vi "Aquisição.vi"(8 "error in (no error)":errorcluster, 10 "rt fifo":refnum<k33>, 11 "FPGA VI Reference In":refnum<k20>) -> (0 "error out":errorcluster, 2 "rt fifo 2":refnum<k33>, 3 "FPGA VI Reference Out":refnum<k20>)   [LabVIEW 2013]
uses:
  PRBScontrol.ctl
  <vilib>/Platform/TimedLoop/XDataNode/timing_clust.ctl
  <vilib>/Platform/TimedLoop/XDataNode/nitl_modes.ctl
  <vilib>/Platform/TimedLoop/XDataNode/wakeup.ctl
  PRBSparameters.ctl
  <vilib>/rvi/interface/common/niFpgaWaitOnOcc.vi
  <vilib>/Utility/error.llb/Error Cluster From Error Code.vi
  <vilib>/rvi/errors/niLvFpgaAdjustHostInterfaceError.vi
  <vilib>/Platform/TimedLoop/XDataNode/XDataNode.xnode
  <vilib>/rvi/interface/nirviReadWriteControl/nirviReadWriteControl.xnode
  <vilib>/Platform/TimedLoop/XDataNode/XDNodeRunTimeDep.lvlib
  NiFpgaLv.dll
  <vilib>/rvi/interface/Simulation/niFpgaSimulationCallBeginRW.vi
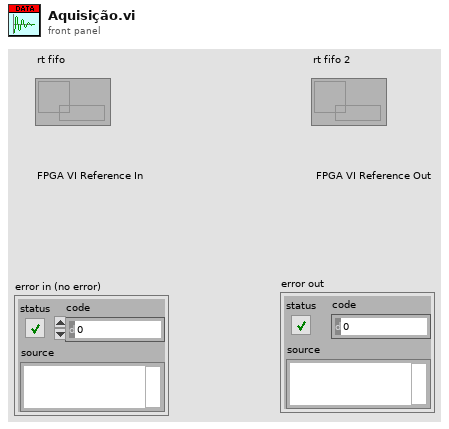
[diagram p1: front panel]
types:
  T1 = typedef "PRBScontrol.ctl" = enum16{"Create", "Get data point"}
  T2 = typedef "XDNodeRunTimeDep.lvlib/timing_clust.ctl" = cluster{"Expected End [f-1]":u64, "Actual End [f-1]":u64, "Finished Late? [f-1]":bool, "Expected End [i-1]":u64, "Actual End [i-1]":u64, "Finished Late? [i-1]":bool, "Expected Start [i]":u64, "Actual Start [i]":u64, "Expected Start [f]":u64, "Actual Start [f]":u64, "Source Name":string, "Structure Name":string, "Period":i64, "Deadline":i64, "Offset":i64, "Start":i64, "Priority":i32, "Timeout":i32, "Mode":T3, "Wakeup Reason":T4, "Error":errorcluster, "Source Type":string, "Secondary Source Type":string, "Global End Time":u64, "Global Start Time":u64, "Frame Duration":u64, "Iteration Duration":u64, "Assigned CPU":i32, "I/O Scan Engine Mode":u32}
  T3 = typedef "XDNodeRunTimeDep.lvlib/nitl_modes.ctl" = enum32{"No Change", "Process missed periods, maintain original phase", "Discard missed periods, maintain original phase", "Process missed periods, ignore original phase", "Discard missed periods, ignore original phase"}
  T4 = typedef "XDNodeRunTimeDep.lvlib/wakeup.ctl" = enum32{"Normal", "Aborted", "Asynchronous wakeup", "Timing source error", "Timed loop error", "Timeout"}
  T5 = typedef "PRBSparameters.ctl" = cluster{"seed":i64, "samples":i64, "upsampling factor":i32, "polynomial order":i32}[]
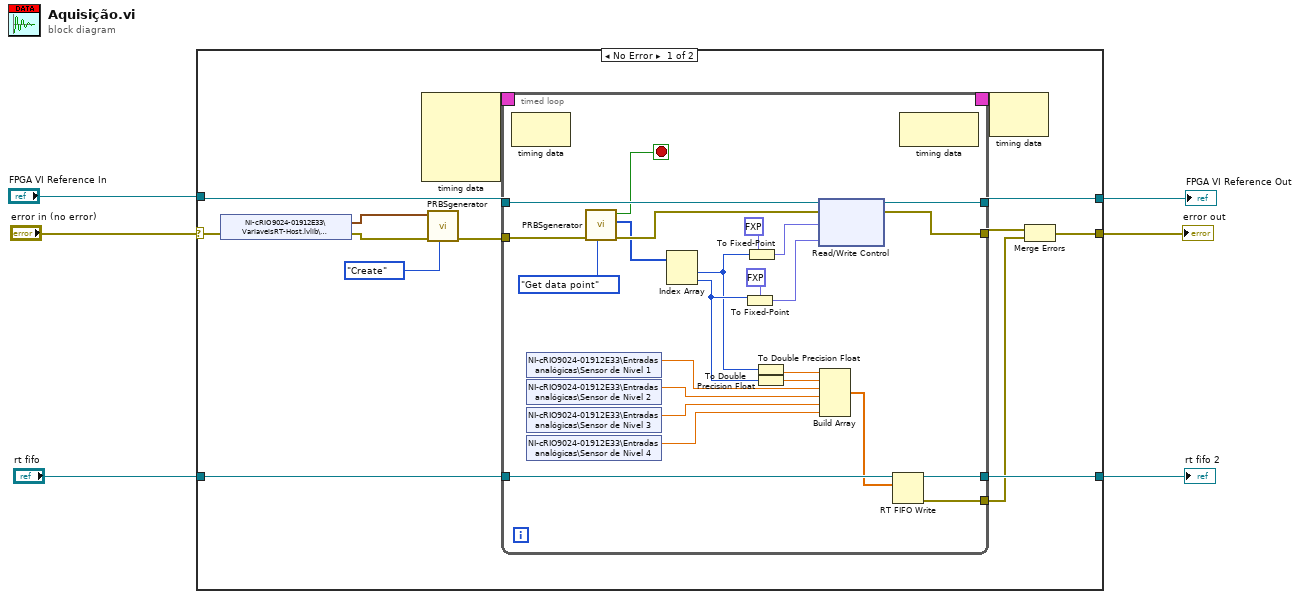
[diagram p0: block diagram]
diagram:
  n1 = case shown="No Error" "error in (no error)" {
    selector: "error in (no error)" -> [w17 w50]
    tunnel: "FPGA VI Reference In" -> [w18 w51]
    tunnel: [w16 w51] -> w3
    tunnel: [w11 w50] -> w5
    tunnel: "rt fifo" -> [w15 w49]
    tunnel: [w14 w49] -> w1
    frame No Error {
      n2 = shared-variable "NI-cRIO9024-01912E33\\VariaveisRT-Host.lvlib\\PRBSparameters"(error in=w17) -> (w7:T5, error out=w8:errorcluster)
      n3 = node-c288() -> (w20:T2)  [unwired: 4 in]
      n4 = call "PRBSgenerator.vi"("Action"=PRBScontrol."Create", "error in (no error)"=w8, "PRBS Parameters"=w7) -> ("error out"=w9:errorcluster)  [unwired: 6 in, 2 out]
      n5 = timed-loop {
        timing: w20 -> [_]
        timing-out: [_] -> w19
        tunnel: w15 -> [w44]
        tunnel: [w38] -> w14
        tunnel: [w37] -> w12
        tunnel: w18 -> [w29]
        tunnel: w9 -> [w36]
        tunnel: [w27] -> w16
        tunnel: [w26] -> w13
        stop <- w22 stop-if-true
        n6 = node-c288() -> ()  [unwired: 1 in, 1 out]
        n7 = shared-variable "NI-cRIO9024-01912E33\\Entradas analógicas\\Sensor de Nivel 1"() -> (w43:dbl)  [unwired: 1 in, 1 out]
        n8 = shared-variable "NI-cRIO9024-01912E33\\Entradas analógicas\\Sensor de Nivel 2"() -> (w42:dbl)  [unwired: 1 in, 1 out]
        n9 = shared-variable "NI-cRIO9024-01912E33\\Entradas analógicas\\Sensor de Nivel 3"() -> (w41:dbl)  [unwired: 1 in, 1 out]
        n10 = shared-variable "NI-cRIO9024-01912E33\\Entradas analógicas\\Sensor de Nivel 4"() -> (w40:dbl)  [unwired: 1 in, 1 out]
        n11 = call "PRBSgenerator.vi"("Action"=PRBScontrol."Get data point", "error in (no error)"=w36) -> ("error out"=w28:errorcluster, "PRBS out"=w23:u8[], "Finalizado?"=w22:bool)  [unwired: 7 in]
        n12 = Index Array(array=w23) -> (element #1=w30:u8, element #2=w31:u8)  [unwired: 2 in]
        n13 = To Fixed-Point(fixed-point type=fxp<+/-,20,5> 0.0, number=w31) -> (fixed-point=w25:fxp<+/-,20,5>)
        n14 = To Fixed-Point(fixed-point type=fxp<+/-,20,5> 0.0, number=w30) -> (fixed-point=w24:fxp<+/-,20,5>)
        n15 = To Double Precision Float(number=w30) -> (double precision float=w32:dbl)
        n16 = To Double Precision Float(number=w31) -> (double precision float=w33:dbl)
        n17 = xnode "Read/Write Control"("FPGA VI Reference In"=w29, "error in"=w28, "Bomba 1"=w24, "Bomba 2"=w25) -> ("FPGA VI Reference Out"=w27:refnum<k20>, "error out"=w26:errorcluster)
        n18 = Build Array(w32, w33, w43, w42, w41, w40) -> (w39:dbl[])
        n19 = RT FIFO Write(0:w44, 1:w39) -> (8:w38:refnum<k33>, 11:w37:errorcluster)  [unwired: 3 in, 2 out]
        n20 = node-c288() -> ()  [unwired: 1 in, 1 out]
      }
      n21 = node-c288(w19) -> ()  [unwired: 1 out]
      n22 = Merge Errors(w13, w12) -> (w11:errorcluster)
    }
    frame Error {
    }
  }
  "error out" <- w5
  "FPGA VI Reference Out" <- w3
  "rt fifo 2" <- w1
